vi "determineNewLogFilePath.vi"(8 "error in (no error)":errorcluster, 11 "Logger in":refnum<class "Log.lvclass">) -> (0 "error out":errorcluster, 2 "logFilePath":path, 3 "Logger out":refnum<class "Log.lvclass">)   [LabVIEW 2013, in "Log.lvclass"]
uses:
  Log.lvclass
  Log.lvclass/Log.ctl
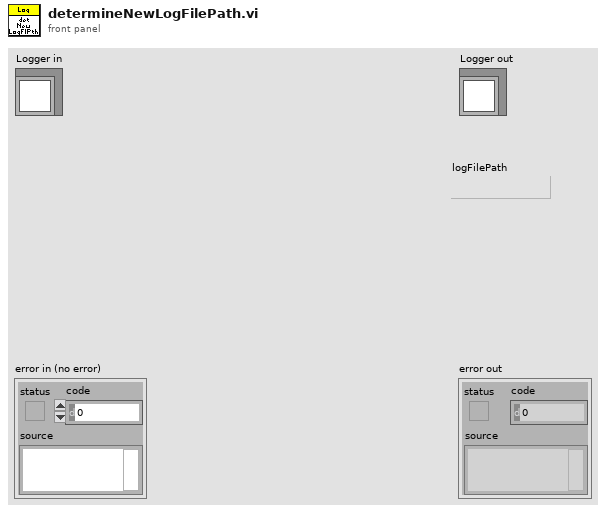
[diagram p1: front panel]
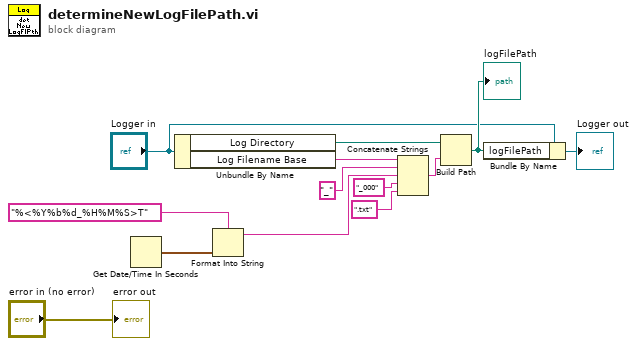
[diagram p0: block diagram]
diagram:
  n1 = Get Date/Time In Seconds() -> (seconds since 1Jan1904=w8:timestamp)
  n2 = Unbundle By Name("Logger in") -> ("Log Directory"=w3:path, "Log Filename Base"=w1:string)
  n3 = Format Into String(format string="%<%Y%b%d_%H%M%S>T", w8) -> (resulting string=w11:string)  [unwired: 2 in, 1 out]
  n4 = Concatenate Strings(w1, "_" ("string"), w11, "_000" ("string"), ".txt" ("string")) -> (w9:string)
  n5 = Build Path(base path=w3, name or relative path=w9) -> (appended path=w5:path)
  "logFilePath" <- w5
  n6 = Bundle By Name(cluster="Logger in", "logFilePath"=w5) -> (→"Logger out":refnum<class "Log.lvclass">)
  "error out" <- "error in (no error)"
